vi "Periodic Tasks.vi"(8 "error in":errorcluster) -> ()   [LabVIEW 2011]
doc: "This VI runs in parallel to other tasks. It can contain as many user-defined periodic loops as you need. These can carry out PID or other sorts of timed response."
uses:
  <vilib>/Rock Robotics/SystemInterfaces/Utilities/FPGA_UtilitiesLED State.ctl
  <vilib>/Rock Robotics/SystemInterfaces/Utilities/FPGA_UtilitiesLED Source.ctl
  Robot Global Data.vi
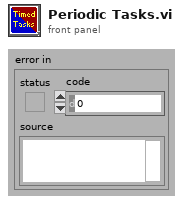
[diagram p1: front panel]
types:
  T1 = typedef "WPI_GyroDevRef.ctl" = cluster{"DevStatus":errorcluster, "Analog Module":T2, "Analog Channel":T3, "Offset":dbl, "Gain (VoltsPerDegree/Second)":dbl}
  T2 = typedef "FPGA_TypedefAnalogModule.ctl" = enum16{"Analog Module 1", "Analog Module 2"}
  T3 = typedef "FPGA_AIChannel.ctl" = enum8{"AI 1", "AI 2", "AI 3", "AI 4", "AI 5", "AI 6", "AI 7", "AI 8", "Invalid"}
  T4 = typedef "WPI_DigitalInputDevRef.ctl" = cluster{"DevStatus":errorcluster, "DIO Channel":T5, "Digital Module":T6}
  T5 = typedef "FPGA_DIOChannel.ctl" = enum8{"DIO 1", "DIO 2", "DIO 3", "DIO 4", "DIO 5", "DIO 6", "DIO 7", "DIO 8", "DIO 9", "DIO 10", "DIO 11", "DIO 12", "DIO 13", "DIO 14", "Invalid"}
  T6 = typedef "FPGA_TypedefDigitalModule.ctl" = enum16{"Digital Module 1", "Digital Module 2"}
  T7 = typedef "WPI_AnalogChannelDevRef.ctl" = cluster{"DevStatus":errorcluster, "Analog Module":T2, "Analog Channel":T3}
  T8 = typedef "WPI_JoystickDevRef.ctl" = cluster{"Device":T9}
  T9 = typedef "WPI_JoystickDeviceEnum.ctl" = enum16{"USB 1", "USB 2", "USB 3", "USB 4", "Kinect 1", "Kinect 2"}
  T10 = typedef "WPI_RobotDriveDevRef.ctl" = cluster{"DevStatus":errorcluster, "Motors[]":T11[], "Square Inputs":bool, "Max Output":dbl, "Isochronous":bool}
  T11 = typedef "WPI_MotorControlDeviceRef.ctl" = cluster{"DeviceStatus":errorcluster, "Type":enum16{"PWM", "CAN"}, "PWM":cluster{"Digital Module":T6, "PWM Channel":T12, "DeadBand":T13}, "CAN":cluster{"Device Number":u8, "Control Mode":T14, "Semaphore":T15, "Max Vout":dbl}, "Invert":bool, "TransformRef":T16, "InvTransformRef":T16}
  T12 = typedef "FPGA_DIOPWMChannel.ctl" = enum8{"PWM 1", "PWM 2", "PWM 3", "PWM 4", "PWM 5", "PWM 6", "PWM 7", "PWM 8", "PWM 9", "PWM 10", "Invalid"}
  T13 = typedef "WPI_PWMDeadband.ctl" = cluster{"Name":string, "maxPositivePwm":i32, "minPositivePwm":i32, "centerPwm":i32, "maxNegativePwm":i32, "minNegativePwm":i32, "angularRange":u16}
  T14 = typedef "WPI_CANJaguar_ControlMode.ctl" = enum8{"Percent VBus", "Current", "Speed", "Position", "Voltage"}
  T15 = typedef "Semaphore RefNum" = refnum<k1>
  T16 = typedef "WPI_PWMTransform_ConPane.ctl" = refnum<vi>
  T17 = cluster{"JoystickDevRef":T8, "RobotDriveDevRef":T10, "GyroDevRef":T1, "GyroDevRef":T1, "AIDeviceRef":T7, "AIDeviceRef":T7, "DigitalInputDevRef":T4, "DigitalInputDevRef":T4, "DigitalInputDevRef":T4, "DigitalInputDevRef":T4}
  T18 = typedef "FPGA_UtilitiesLED State.ctl" = enum16{"Off", "On", "Toggle"}
  T19 = typedef "FPGA_UtilitiesLED Source.ctl" = enum16{"User LED", "FPGA LED"}
  T20 = typedef "WPI_CompressorDevRef.ctl" = cluster{"DevStatus":errorcluster, "DigitalInputDevRef":T4, "RelayDevRef":T21}
  T21 = typedef "WPI_RelayDevRef.ctl" = cluster{"DevStatus":errorcluster, "Relay Channel":T22, "Digital Module":T6, "Relay Direction":T23}
  T22 = typedef "FPGA_DIORelayChannel.ctl" = enum8{"Relay 1", "Relay 2", "Relay 3", "Relay 4", "Relay 5", "Relay 6", "Relay 7", "Relay 8", "Invalid"}
  T23 = typedef "WPI_RelayDirection.ctl" = enum16{"Both directions", "Forward only", "Reverse only"}
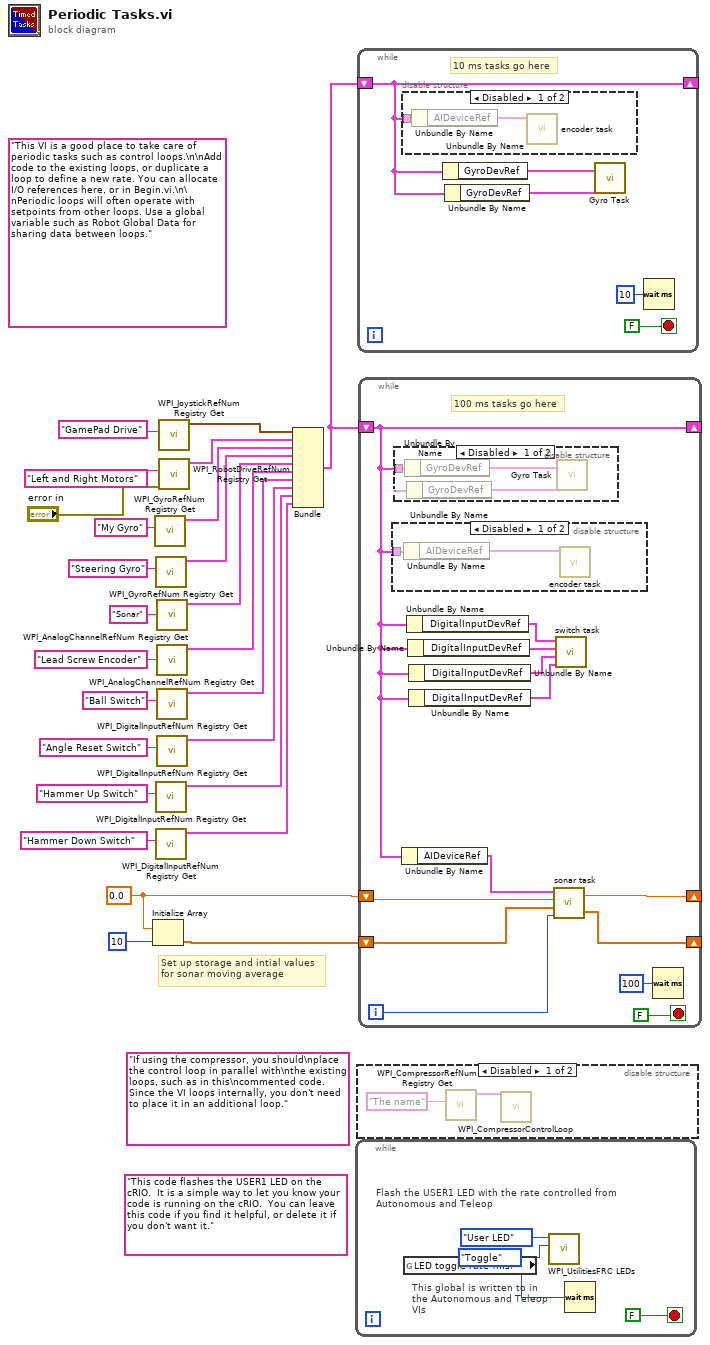
[diagram p0: block diagram]
diagram:
  w2 = 0.0 ("y")
  (unwired) "If using the compressor, you should\nplace the control loop in parallel with\nthe existing loops, such as in this\ncommented code. Since the VI loops internally, you don't need to place it in an additional loop."
  (unwired) "This code flashes the USER1 LED on the cRIO.  It is a simple way to let you know your code is running on the cRIO.  You can leave this code if you find it helpful, or delete it if you don't want it."
  (unwired) "This VI is a good place to take care of periodic tasks such as control loops.\n\nAdd code to the existing loops, or duplicate a loop to define a new rate. You can allocate I/O references here, or in Begin.vi.\n\nPeriodic loops will often operate with setpoints from other loops. Use a global variable such as Robot Global Data for sharing data between loops."
  # "Set up storage and intial values\nfor sonar moving average"
  n1 = Initialize Array(w2, 10 ("Average")) -> (w1:dbl[])
  n2 = call <vilib>:"WPI_GyroRefNum Registry Get.vi"("refnum name"="My Gyro") -> ("GyroDevRef"=w18:T1)  [unwired: 9 in, 1 out]
  n3 = call <vilib>:"WPI_GyroRefNum Registry Get.vi"("refnum name"="Steering Gyro") -> ("GyroDevRef"=w12:T1)  [unwired: 9 in, 1 out]
  n4 = call <vilib>:"WPI_DigitalInputRefNum Registry Get.vi"("refnum name"="Hammer Up Switch") -> ("DigitalInputDevRef"=w5:T4)  [unwired: 9 in, 1 out]
  n5 = call <vilib>:"WPI_DigitalInputRefNum Registry Get.vi"("refnum name"="Hammer Down Switch") -> ("DigitalInputDevRef"=w4:T4)  [unwired: 9 in, 1 out]
  n6 = call <vilib>:"WPI_AnalogChannelRefNum Registry Get.vi"("refnum name"="Sonar") -> ("AIDeviceRef"=w13:T7)  [unwired: 9 in, 1 out]
  n7 = call <vilib>:"WPI_AnalogChannelRefNum Registry Get.vi"("refnum name"="Lead Screw Encoder") -> ("AIDeviceRef"=w14:T7)  [unwired: 9 in, 1 out]
  n8 = call <vilib>:"WPI_DigitalInputRefNum Registry Get.vi"("refnum name"="Ball Switch") -> ("DigitalInputDevRef"=w10:T4)  [unwired: 9 in, 1 out]
  n9 = call <vilib>:"WPI_DigitalInputRefNum Registry Get.vi"("refnum name"="Angle Reset Switch") -> ("DigitalInputDevRef"=w8:T4)  [unwired: 9 in, 1 out]
  n10 = call <vilib>:"WPI_JoystickRefNum Registry Get.vi"("refnum name"="GamePad Drive") -> ("JoystickDevRef"=w23:T8)  [unwired: 1 in, 9 out]
  n11 = call <vilib>:"WPI_RobotDriveRefNum Registry Get.vi"("error in (no error)"="error in", "refnum name"="Left and Right Motors") -> ("RobotDriveDevRef"=w22:T10)  [unwired: 9 out]
  n12 = Bundle("JoystickDevRef"=w23, "RobotDriveDevRef"=w22, "GyroDevRef"=w18, "GyroDevRef"=w12, "AIDeviceRef"=w13, "AIDeviceRef"=w14, "DigitalInputDevRef"=w10, "DigitalInputDevRef"=w8, "DigitalInputDevRef"=w5, "DigitalInputDevRef"=w4) -> (w21:T17)  [unwired: 1 out]
  n13 = while {
    stop <- FALSE stop-if-true
    # "This global is written to in the Autonomous and Teleop VIs"
    # "Flash the USER1 LED with the rate controlled from Autonomous and Teleop"
    n14 = global read "Robot Global Data.vi" "LED toggle rate (ms)"() -> (w26:u32)
    n15 = call <vilib>:"WPI_UtilitiesFRC LEDs.vi"("State"=FPGA_UtilitiesLED_State."Toggle", "LED Type"=FPGA_UtilitiesLED_Source."User LED") -> ()  [unwired: 1 in, 9 out]
    n16 = Wait (ms)(milliseconds to wait=w26) -> ()  [unwired: 1 out]
  }
  n17 = while {
    shift-right: [w30] -> _
    shift-left: w21 -> [w30]
    stop <- FALSE stop-if-true
    # "10 ms tasks go here"
    n18 = disable-structure shown="Disabled" {
      disable-tunnel: w30 -> [w35 _]
      frame Disabled {
        n19 = Unbundle By Name(w35) -> ("AIDeviceRef"=w36:T7)
        n20 = call "encoder task.vi"("AIDeviceRef"=w36) -> ()  [unwired: 11 in]
      }
      frame Enabled {
      }
    }
    n21 = Unbundle By Name(w30) -> ("GyroDevRef"=w32:T1)
    n22 = Unbundle By Name(w30) -> ("GyroDevRef"=w31:T1)
    n23 = call "Gyro Task.vi"("GyroDevRef"=w32, "GyroDevRef 2"=w31) -> ()  [unwired: 4 in]
    n24 = Wait (ms)(milliseconds to wait=u32 10) -> ()  [unwired: 1 out]
  }
  n25 = disable-structure shown="Disabled" {
    frame Disabled {
      n26 = call <vilib>:"WPI_CompressorRefNum Registry Get.vi"("refnum name"="The name") -> ("CompressorDevRef"=w38:T20)  [unwired: 9 in, 1 out]
      n27 = call <vilib>:"WPI_CompressorControlLoop.vi"("CompressorDevRef"=w38) -> ()  [unwired: 11 in]
    }
    frame Enabled {
    }
  }
  n28 = while {
    shift-right: [w46] -> _
    shift-left: w21 -> [w46]
    shift-right: [w39] -> _
    shift-left: w1 -> [w42]
    shift-right: [w40] -> _
    shift-left: w2 -> [w43]
    i -> [w41]
    stop <- FALSE stop-if-true
    # "100 ms tasks go here"
    n29 = disable-structure shown="Disabled" {
      disable-tunnel: w46 -> [w52 _]
      frame Disabled {
        n30 = Unbundle By Name(w52) -> ("AIDeviceRef"=w53:T7)
        n31 = call "encoder task.vi"("AIDeviceRef"=w53) -> ()  [unwired: 11 in]
      }
      frame Enabled {
      }
    }
    n32 = disable-structure shown="Disabled" {
      disable-tunnel: w46 -> [w54 _]
      frame Disabled {
        n33 = Unbundle By Name(w54) -> ("GyroDevRef"=w56:T1)
        n34 = Unbundle By Name(w54) -> ("GyroDevRef"=w55:T1)
        n35 = call "Gyro Task.vi"("GyroDevRef"=w56, "GyroDevRef 2"=w55) -> ()  [unwired: 4 in]
      }
      frame Enabled {
      }
    }
    n36 = Unbundle By Name(w46) -> ("AIDeviceRef"=w49:T7)
    n37 = Unbundle By Name(w46) -> ("DigitalInputDevRef"=w48:T4)
    n38 = Unbundle By Name(w46) -> ("DigitalInputDevRef"=w47:T4)
    n39 = Unbundle By Name(w46) -> ("DigitalInputDevRef"=w45:T4)
    n40 = Unbundle By Name(w46) -> ("DigitalInputDevRef"=w44:T4)
    n41 = call "sonar task.vi"("i"=w41, "Array In"=w42, "Sum In"=w43, "AIDeviceRef"=w49) -> ("Array Out"=w39:dbl[], "Sum Out"=w40:dbl)
    n42 = call "switch task.vi"("DigitalInputDevRef 4"=w44, "DigitalInputDevRef 3"=w45, "DigitalInputDevRef 2"=w47, "DigitalInputDevRef"=w48) -> ()  [unwired: 1 in]
    n43 = Wait (ms)(milliseconds to wait=u32 100) -> ()  [unwired: 1 out]
  }
